vi "Init_Test.vi"(8 "error in (no error)":errorcluster caption="entrée d'erreur (pas d'erreur)", 11 "Generate_SN en entrée":refnum<class "Generate_ID_Product_Nodon.lvclass">) -> (0 "error out":errorcluster caption="sortie d'erreur", 3 "Generate_SN en sortie":refnum<class "Generate_ID_Product_Nodon.lvclass">)   [LabVIEW 2020, in "Library Test.lvlib" / "Generate_ID_Product_Nodon.lvclass"]
uses:
  Generate_ID_Product_Nodon.lvclass
  C:/Users/ngarcin/OneDrive - Altyor/Standard TB/Class/Test/Test (Default)/Test (Default).lvclass
  Commun VI/TypeDef/Commande Test/Commande Type Test.ctl
  Test_Without_Instr/Test_Without_Inst.lvclass
  Generate_ID_Product_Nodon.lvclass/Generate_ID_Product_Nodon.ctl
  Commun VI/Library Commun.lvlib
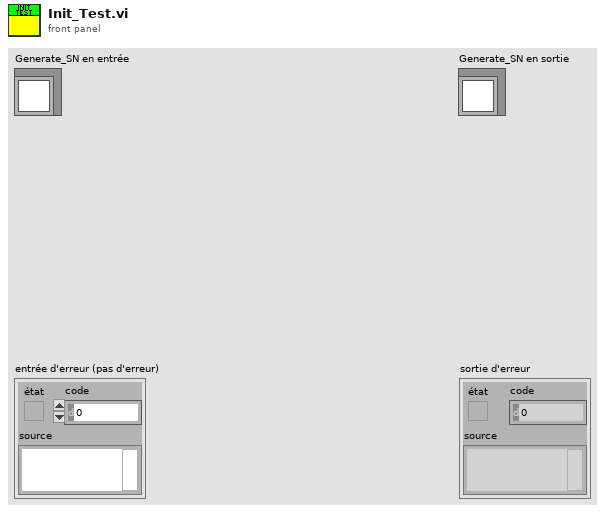
[diagram p1: front panel]
types:
  T1 = typedef "Library Commun.lvlib/Commande Type Test.ctl" = enum16{"Function", "Test", "Calculation"}
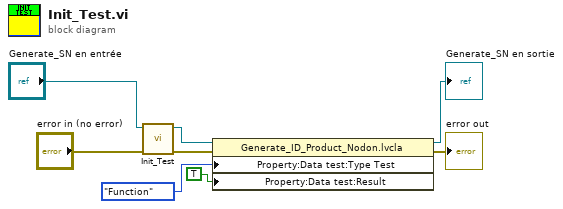
[diagram p0: block diagram]
diagram:
  n1 = call-parent "Init_Test.vi"("error in (no error)"="error in (no error)", "Test_Without_Inst en entrée"="Generate_SN en entrée") -> ("error out"=w6:errorcluster, "Test_Without_Inst en sortie"=w5:refnum<class "Generate_ID_Product_Nodon.lvclass">)  [unwired: 8 in]
  n2 = property class="Generate_ID_Product_Nodon.lvcla"(reference=w5, error in=w6, "Property:Data test:Type Test"=Commande_Type_Test."Function" ("Type Test"), "Property:Data test:Result"=TRUE ("Result")) -> (reference out=→"Generate_SN en sortie":refnum<class "Generate_ID_Product_Nodon.lvclass">, error out=→"error out":errorcluster)
